vi "FUG-HCN.destructor.vi"(0 "i ref in":refnum<vi>, 5 "error in(no error)":errorcluster) -> (19 "error out":errorcluster)   [LabVIEW 2014, in "FUG-HCN.lvlib"]
doc: "This is the destructor of a class.\n\nLicense Agreement for this software:\n\nCopyright (C)\nGesellschaft für Schwerionenforschung, GSI\nPlanckstr. 1\n64291 Darmstadt\nGermany\n\nContact: D.Beck@gsi.de \n\nThis program is free software; you can redistribute it and/or modify it under the terms of the \nGNU General Public License as published by the Free Software Foundation; either version 2 of \nthe license, or (at your option) any later version.\n\nThis program is distributed in the hope that it will be useful, but WITHOUT ANY WARRANTY; \nwithout even the implied warranty of MERCHANTABILITY or FITNESS FOR A PARTICULAR PURPOSE. See the GNU General License for more details (http://www.gnu.org).\n\nGesellschaft für Schwerionenforschung, GSI\nPlanckstr. 1, 64291 Darmstadt, Germany\nFor all questions and ideas contact: M.Richter@gsi.de, H.Brand@gsi.de or D.Beck@gsi.de.\nLast update: 16-JUN-2004"
uses:
  FUG-HCN.lvlib
  CS_Core/BaseProcess/BaseProcess.lvlib
  CSlibraries-extern/DimLVEvent/LVDimInterface/LVDimInterface.lvlib
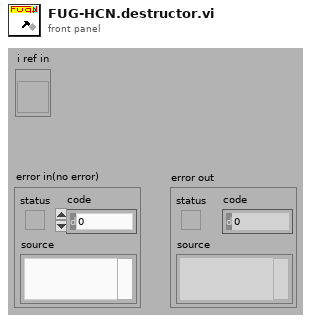
[diagram p1: front panel]
types:
  T1 = enum16{"SetAttribute", "GetAttribute", "CreateAttribute", "DestroyAttribute", "DestroyAllAtributes"}
  T2 = typedef "FUG-HCN.lvlib/FUG-HCN.i attribute.ctl" = cluster{"SetStatus":bool, "Set Voltage":dbl, "Nom Voltage":dbl, "VoltageID":i32, "CurrentID":i32}
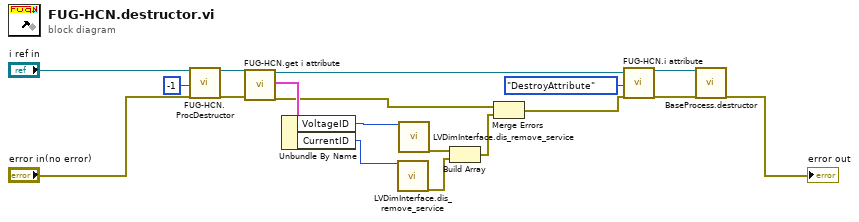
[diagram p0: block diagram]
diagram:
  n1 = call "FUG-HCN.ProcDestructor.vi"("i ref in"="i ref in", "ms timeout (100)"=-1, "error in (no error)"="error in(no error)") -> ("i ref out"=w11:refnum<vi>, "error out"=w10:errorcluster)  [unwired: 14 in, 1 out]
  n2 = call "FUG-HCN.get i attribute.vi"("i ref in"=w11, "error in (no error)"=w10) -> ("i ref out"=w8:refnum<vi>, "i attribute"=w9:T2, "error out"=w2:errorcluster)  [unwired: 15 in]
  n3 = Unbundle By Name(w9) -> ("VoltageID"=w7:i32, "CurrentID"=w6:i32)
  n4 = call "LVDimInterface.dis_remove_service.vi"("my_serviceID"=w6) -> ("error out"=w4:errorcluster)  [unwired: 18 in]
  n5 = call "LVDimInterface.dis_remove_service.vi"("my_serviceID"=w7) -> ("error out"=w5:errorcluster)  [unwired: 18 in]
  n6 = Build Array(w5, w4) -> (w3:errorcluster[])
  n7 = Merge Errors(w2, w3) -> (w1:errorcluster)
  n8 = call "FUG-HCN.i attribute.vi"("VI Refnum"=w8, "Action"=T1."DestroyAttribute", "error in (no error)"=w1) -> ("VI Refnum out"=w17:refnum<vi>, "error out"=w16:errorcluster)  [unwired: 14 in, 1 out]
  n9 = call "BaseProcess.destructor.vi"("i ref in"=w17, "error in (no error)"=w16) -> ("error out"=→"error out":errorcluster)  [unwired: 17 in]
